vi "File_Segment File.vi"(8 "current time in":timestamp, 9 "path in":path, 10 "Segment by":T1=enum."Size (MB)", 11 "Segment Every":dbl) -> (3 "Boolean":bool)   [LabVIEW 2023, in "File.lvclass"]
doc: "Determines based on the parameters whether the segmentation conditions have been met."
uses:
  File.lvclass
  SegmentationOptions.ctl
panel:
  out "error out":errorcluster
  in  "error in (no error)":errorcluster
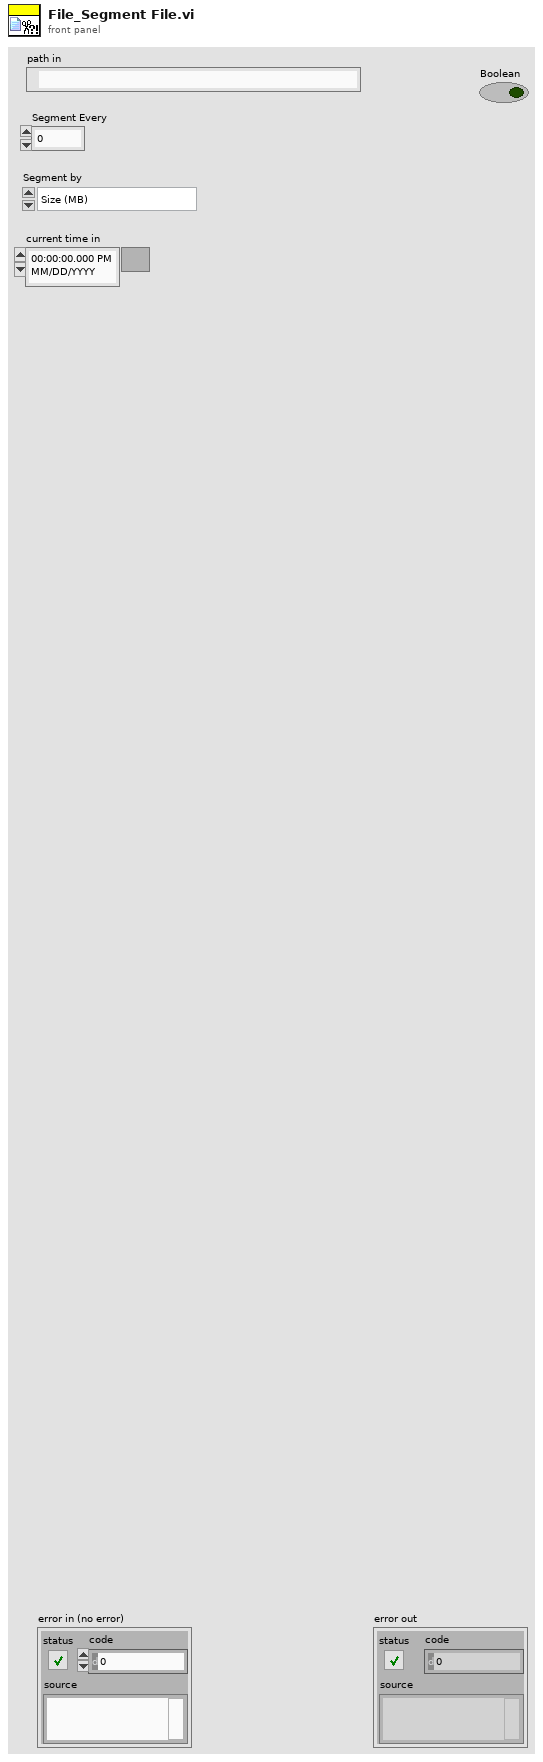
[diagram p1: front panel]
types:
  T1 = typedef "SegmentationOptions.ctl" = enum16{"Time (s)", "Size (MB)"}
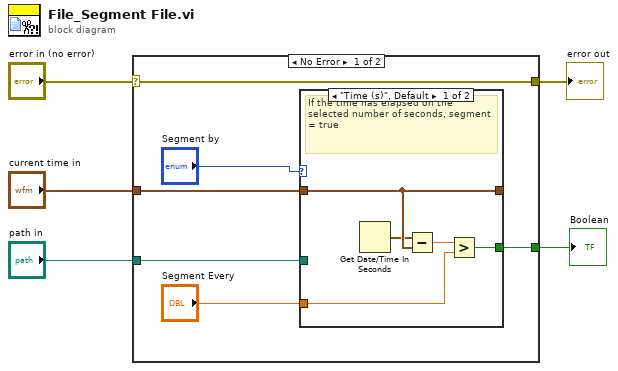
[diagram p0: block diagram]
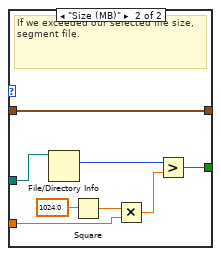
[diagram p2: hidden frame]
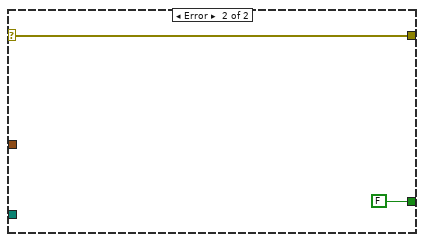
[diagram p3: hidden frame]
diagram:
  n1 = case shown="No Error" "error in (no error)" {
    selector: "error in (no error)" -> [w10 w26]
    tunnel: [w7 FALSE] -> w2
    tunnel: "current time in" -> [w11 _]
    tunnel: [w10 w26] -> w4
    tunnel: "path in" -> [w9 _]
    frame No Error {
      n2 = case shown="\"Time (s)\", Default" "Segment by" {
        tunnel: "Segment Every" -> [w12 w20]
        tunnel: [w16 w22] -> w7
        tunnel: w11 -> [w15 w21]
        tunnel: [w15 w21] -> _
        tunnel: w9 -> [_ w18]
        frame "Time (s)", Default {
          # "If the time has elapsed on the selected number of seconds, segment = true"
          n3 = Get Date/Time In Seconds() -> (seconds since 1Jan1904=w14:timestamp)
          n4 = Subtract(x=w14, y=w15) -> (x-y=w13:dbl)
          n5 = Greater?(x=w13, y=w12) -> (0:w16:bool)
        }
        frame "Size (MB)" {
          # "If we exceeded our selected file size, segment file."
          n6 = File/Directory Info(path=w18) -> (size=w17:i64)  [unwired: 1 in, 6 out]
          n7 = Square(x=1024.0) -> (x^2=w23:dbl)
          n8 = Multiply(x=w23, y=w20) -> (x*y=w19:dbl)
          n9 = Greater?(x=w17, y=w19) -> (0:w22:bool)
        }
      }
    }
    frame Error {
    }
  }
  "error out" <- w4
  "Boolean" <- w2
